vi "S2C_LoadScript.vi"(8 "Error In":errorcluster) -> (0 "Error Out":errorcluster)   [LabVIEW 2015]
doc: "Loads the selected script file into the build script table."
uses:
  Globals/S2C_Globals.vi
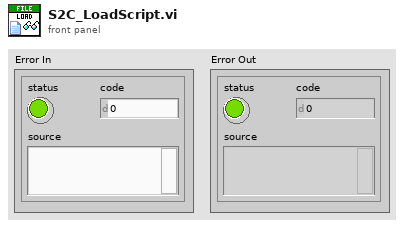
[diagram p1: front panel]
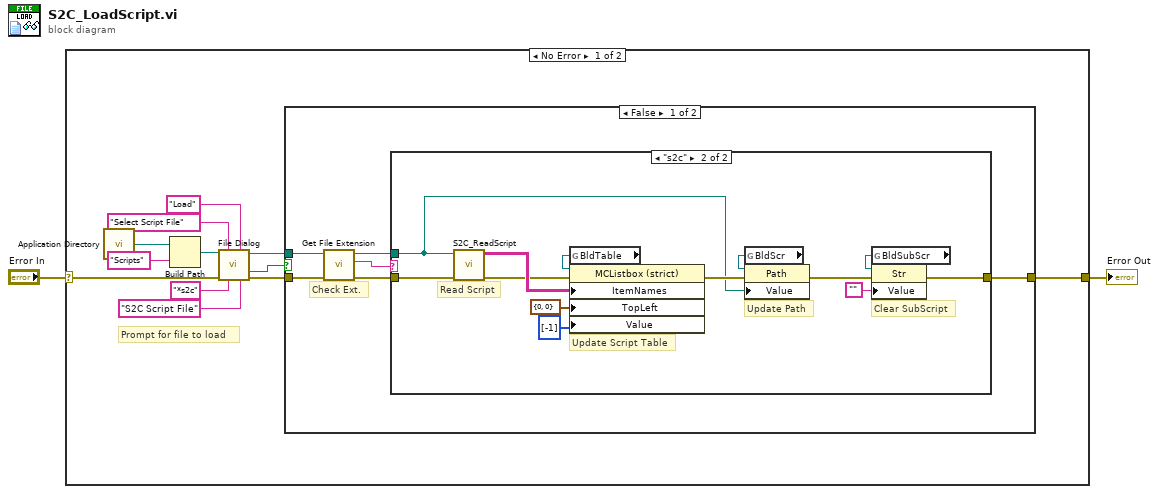
[diagram p0: block diagram]
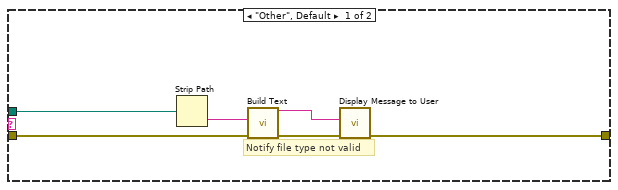
[diagram p2: hidden frame]
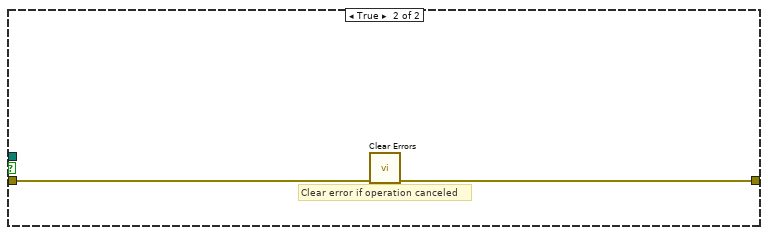
[diagram p3: hidden frame]
diagram:
  n1 = case shown="No Error" "Error In" {
    selector: "Error In" -> [w14 w42]
    tunnel: [w5 w42] -> w1
    frame No Error {
      # "Prompt for file to load"
      n2 = call <vilib>:"Application Directory.vi"() -> ("Application Directory"=w12:path)
      n3 = Build Path(base path=w12, name or relative path="Scripts") -> (appended path=w10:path)
      n4 = call "File Dialog"("start path"=w10, "prompt"="Select Script File", "button label"="Load", "error in"=w14, "pattern (all files)"="*s2c", "pattern label"="S2C Script File") -> ("selected path"=w4:path, "cancelled"=w3:bool, "error out"=w6:errorcluster)  [unwired: 6 in, 1 out]
      n5 = case shown="False" w3 {
        tunnel: w6 -> [w19 w41]
        tunnel: w4 -> [w18 _]
        tunnel: [w20 w40] -> w5
        frame False {
          # "Check Ext."
          n6 = call <vilib>:"Get File Extension.vi"("error in (no error)"=w19, "file"=w18) -> ("error out"=w16:errorcluster, "lowercase file extension"=w15:string, "dup file"=w17:path)  [unwired: 5 in, 2 out]
          n7 = case shown="\"s2c\"" w15 {
            tunnel: [w22 w31] -> w20
            tunnel: w17 -> [w25 w29]
            tunnel: w16 -> [w26 w30]
            frame "Other", Default {
              # "Notify file type not valid"
              n8 = Strip Path(path=w25) -> (name=w24:string)  [unwired: 1 out]
              n9 = call "Build Text"("File"=w24, "error in (no error)"=w26) -> ("Result"=w21:string, "error out"=w23:errorcluster)  [unwired: 12 in]
              n10 = call "Display Message to User"("error in (no error)"=w23, "Message"=w21) -> ("error out"=w22:errorcluster)  [unwired: 8 in, 1 out]
            }
            frame "s2c" {
              # "Read Script"
              # "Update Script Table"
              # "Clear SubScript"
              # "Update Path"
              n11 = call "S2C_ReadScript.vi"("Error In"=w30, "FilePath"=w29) -> ("Error Out"=w27:errorcluster, "Data"=w28:string[][])  [unwired: 8 in]
              n12 = global read "S2C_Globals.vi" "BldTable"() -> (w39:refnum<vi>)
              n13 = property class="MCListbox (strict)"(reference=w39, error in=w27, "ItemNames"=w28, "TopLeft"=cluster{"Row":u32, "Column":u32} {"Row"=0, "Column"=0} ("Top Left Visible Cell"), "Value"=i32[] [-1]) -> (error out=w35:errorcluster)  [unwired: 1 out]
              n14 = global read "S2C_Globals.vi" "BldScr"() -> (w36:refnum<vi>)
              n15 = property class="Path"(reference=w36, error in=w35, "Value"=w29) -> (error out=w32:errorcluster)  [unwired: 1 out]
              n16 = global read "S2C_Globals.vi" "BldSubScr"() -> (w33:refnum<vi>)
              n17 = property class="Str"(reference=w33, error in=w32, "Value"="") -> (error out=w31:errorcluster)  [unwired: 1 out]
            }
          }
        }
        frame True {
          # "Clear error if operation canceled"
          n18 = call <vilib>:"Clear Errors.vi"("error in (no error)"=w41) -> ("error out"=w40:errorcluster)  [unwired: 5 in, 1 out]
        }
      }
    }
    frame Error {
    }
  }
  "Error Out" <- w1
